vi "Service for Authentication.vi"(11 "IoT Session":refnum<class "IoT Session.lvclass">) -> (2 "Service for Authentication":string)   [LabVIEW 2015, in "NI_AWS_IoT.lvlib" / "IoT Session.lvclass"]
uses:
  IoT Session.lvclass
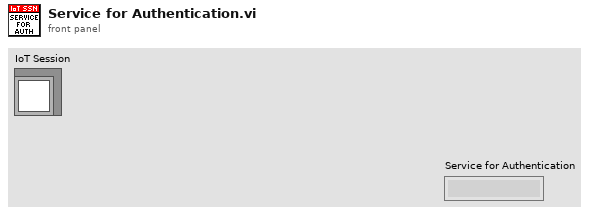
[diagram p1: front panel]
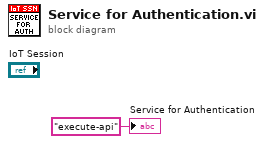
[diagram p0: block diagram]
diagram:
  "Service for Authentication" <- "execute-api" ("Service for Authentication")
